vi "is_empty.vi"(11 "on-board buffer in":T1) -> (2 "is empty?":bool)   [LabVIEW 2010, in "OnBoardBuffer.lvlib"]
uses:
  OnBoardBuffer.lvlib
  OnBoardBuffer.ctl
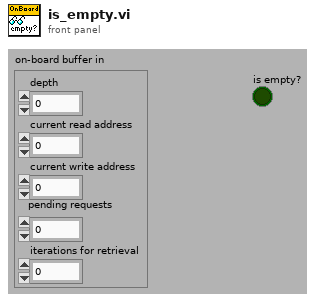
[diagram p1: front panel]
types:
  T1 = typedef "OnBoardBuffer.lvlib/OnBoardBuffer.ctl" = cluster{"depth":u32, "current read address":u32, "current write address":u32, "pending requests":u32, "iterations for retrieval":u32}
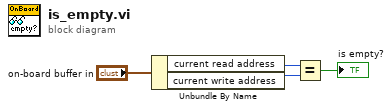
[diagram p0: block diagram]
diagram:
  n1 = Unbundle By Name("on-board buffer in") -> ("current read address"=w3:u32, "current write address"=w2:u32)
  n2 = Equal?(x=w3, y=w2) -> (x = y?=→"is empty?":bool)
